vi "Get Chamber Status-teardown.vi"(5 "Test Error":errorcluster, 6 "Heater State":bool, 7 "Application Exit":bool, 8 "Ramp Rate (deg C / second)":dbl, 9 "Temperature Set Point (deg C)":dbl, 10 "Actual Temperature":dbl, 11 "test case ID":string) -> (3 "result":bool)   [LabVIEW 2018]
doc: "The teardown VI should be executed after the VI under test in the harness VI. In this VI you can evaluate the outputs of the VI under test.\n\nSee the Help Document for more information. (<b>Help</b> > <b>IncQuery Labs</b> > <b>InstaCoverage</b> > <b>InstaCoverage Help...</b>)"
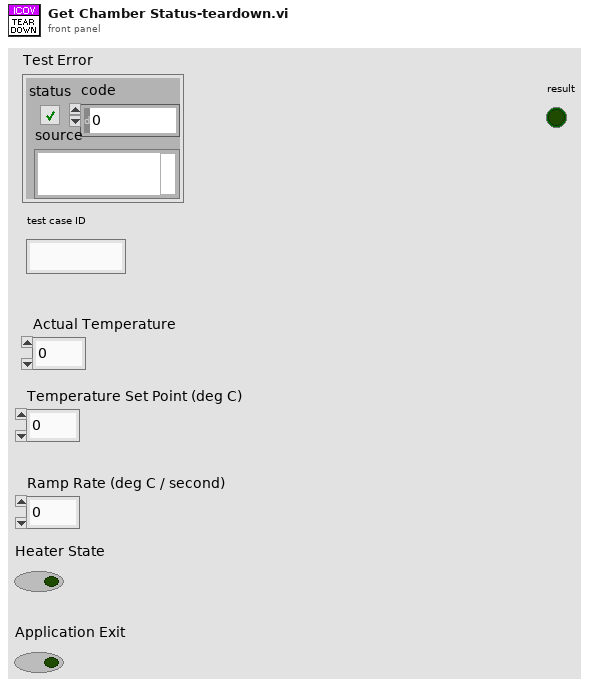
[diagram p1: front panel]
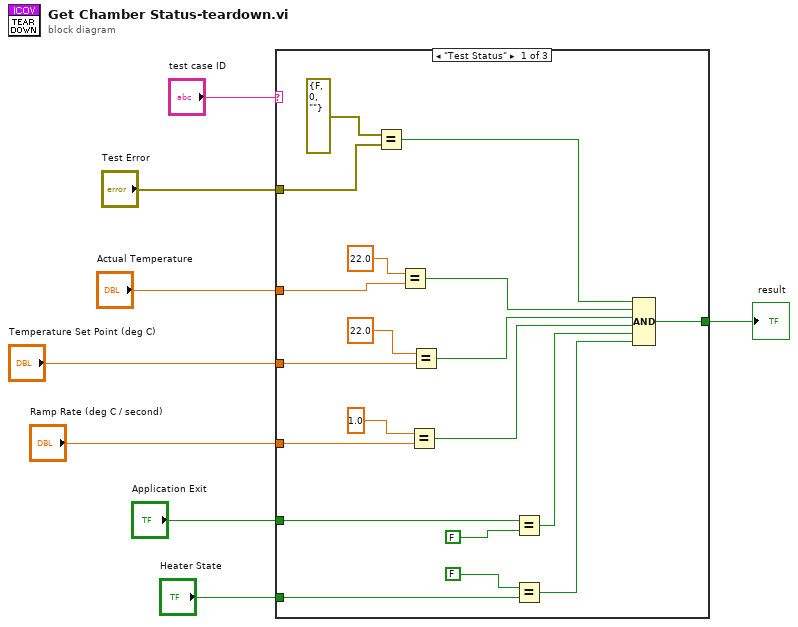
[diagram p0: block diagram]
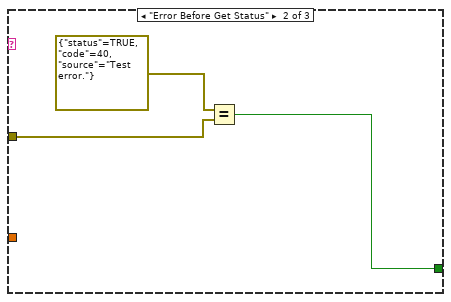
[diagram p2: hidden frame]
diagram:
  n1 = case shown="\"Test Status\"" "test case ID" {
    tunnel: [w11 w28 FALSE] -> w7
    tunnel: "Actual Temperature" -> [w26 _ _]
    tunnel: "Temperature Set Point (deg C)" -> [w24 _ _]
    tunnel: "Ramp Rate (deg C / second)" -> [w22 _ _]
    tunnel: "Application Exit" -> [w21 _ _]
    tunnel: "Heater State" -> [w20 _ _]
    tunnel: "Test Error" -> [w18 w29 _]
    frame "Test Status" {
      n2 = Equal?(x=errorcluster {"status"=FALSE, "code"=0, "source"=""} ("Test Error"), y=w18) -> (x = y?=w10:bool)
      n3 = Equal?(x=22.0, y=w26) -> (x = y?=w9:bool)
      n4 = Equal?(x=1.0, y=w22) -> (x = y?=w14:bool)
      n5 = Equal?(x=22.0, y=w24) -> (x = y?=w15:bool)
      n6 = Equal?(x=w21, y=FALSE) -> (x = y?=w13:bool)
      n7 = Equal?(x=FALSE, y=w20) -> (x = y?=w12:bool)
      n8 = Compound Arithmetic op=AND(w10, w9, w15, w14, w13, w12) -> (w11:bool)
    }
    frame "Error Before Get Status" {
      n9 = Equal?(x=errorcluster {"status"=TRUE, "code"=40, "source"="Test error."} ("Test Error"), y=w29) -> (x = y?=w28:bool)
    }
    frame Default {
    }
  }
  "result" <- w7
